vi "Channel 2.vi"() -> ()   [LabVIEW 2016]
panel:
  in  "Channel Name 2":string="Channel 1"
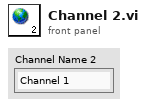
[diagram p1: front panel]
diagram:
